vi "RobotInsideCircleBool.vi"(7 "Ball -> Robot Norm":dbl, 8 "error in (no error)":errorcluster, 9 "Raio":dbl, 10 "Eps":dbl, 11 "KickToSkill in":refnum<class "KickToSkill.lvclass">) -> (0 "error out":errorcluster, 2 "Boolean":bool, 3 "KickToSkill out":refnum<class "KickToSkill.lvclass">)   [LabVIEW 2021, in "KickToSkill.lvclass"]
uses:
  KickToSkill.lvclass
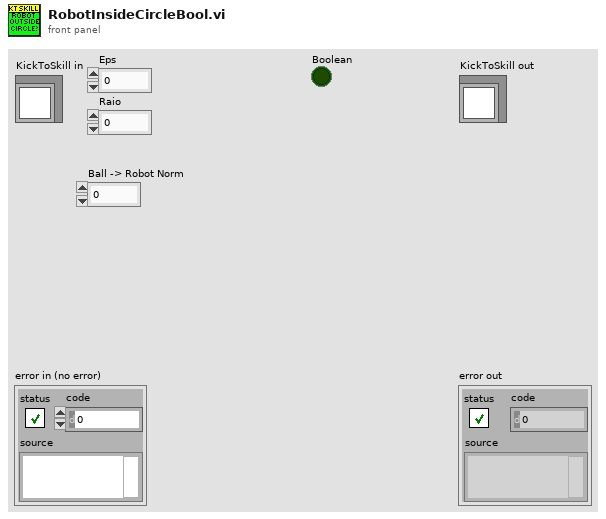
[diagram p1: front panel]
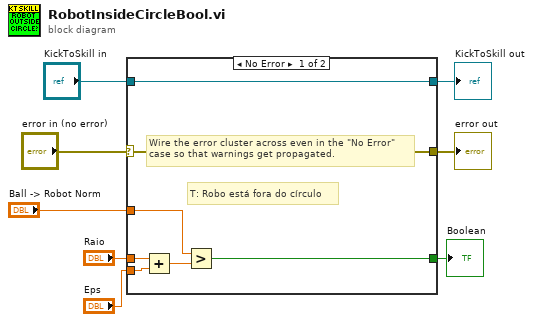
[diagram p0: block diagram]
diagram:
  n1 = case shown="No Error" "error in (no error)" {
    selector: "error in (no error)" -> [w14 w17]
    tunnel: [w14 w17] -> w7
    tunnel: [w15 w16] -> w5
    tunnel: "KickToSkill in" -> [w15 w16]
    tunnel: [w12 _] -> w1
    tunnel: "Ball -> Robot Norm" -> [w11 _]
    tunnel: "Eps" -> [w10 _]
    tunnel: "Raio" -> [w9 _]
    frame No Error {
      # "T: Robo está fora do círculo"
      # "Wire the error cluster across even in the \"No Error\"\ncase so that warnings get propagated."
      n2 = Add(x=w9, y=w10) -> (x+y=w13:dbl)
      n3 = Greater?(x=w11, y=w13) -> (0:w12:bool)
    }
    frame Error {
    }
  }
  "error out" <- w7
  "KickToSkill out" <- w5
  "Boolean" <- w1
